vi "Show Cursors.vi"(6 "Cursor Options":T1={"font"={"Font Name"="Arial", "Size"=14, "Strikeout?"=FALSE, "Italic?"=FALSE, "Underline?"=FALSE, "Outline?"=FALSE, "Shadow?"=FALSE, "Bold?"=FALSE}, "size"=1, "Timestamp"=enum."at TOP", "Vertical Line?"=FALSE, "Horizontal Line?"=FALSE, "alignment(left, top)"={"horizontal"=enum."center", "vertical"=enum."center"}, "TextFormat"="%.3p %.3p %s", "time format (%H:%M:%S)"="%H:%M%:S"} {"size" min=1 max=50}, 8 "error in (no error)":errorcluster, 9 "Coords":T2, 10 "Graph Data":cluster{"Array":dbl[], "Array":dbl[]}[](array[cluster]), 11 "Grapg":refnum<vi>) -> (0 "error out":errorcluster, 3 "output picture":picture)   [LabVIEW 2019]
doc: "Shows real time cursors overlayed in a graph, using just one mouse move event case. The options for the cursors can be highly customized to set up a unique cursor style.\n\nUsage: Place this inside an event structure on any XY graph, in the \"Mouse Move\" event case. Set the options as an input cluster to override the defaults. The output picture control would typically be connected to the XY Graph's \"PlotImages.Front\" property item.\n\nCursor Options\n<b>Horizontal Line?</b> - Draws a horizontal line to intersect each plot\n<b>Verticle Line?</b> - Draws a verticle line at the mouse location to highlight the cursor location (typically on the time scale)\n<b>Timestamp</b> - Sets where to display the timestamp (if you want it at the top or bottom) Used best with the verticle line turned on.\n<b>Font</b> - Setup the font for displaying the cursor text\n<b>Alignment</b> - Sets the alignment options for the text relative to the cursor point\n<b>TextFormat</b> - Sets the text display format at the cursor points to show. Three input parameters are available for the text, which can be accessed using parameter numbers.\ninputs: \n1$ - Timestamp at cursor locations\n2$ - Value of the plot\n3$ - Name of the plot\n\nExamples: $2$.2f\\n\\n%1$s\nThis shows the value of the plot with 2 decimal places. A blank line, then the name of the plot"
uses:
  <vilib>/Utility/miscctls.llb/LVPoint32TypeDef.ctl
  controls/CursorOptions.ctl
panel:
  in  "input picture":picture
  # "%2$.2f\\n\\n%1$s"
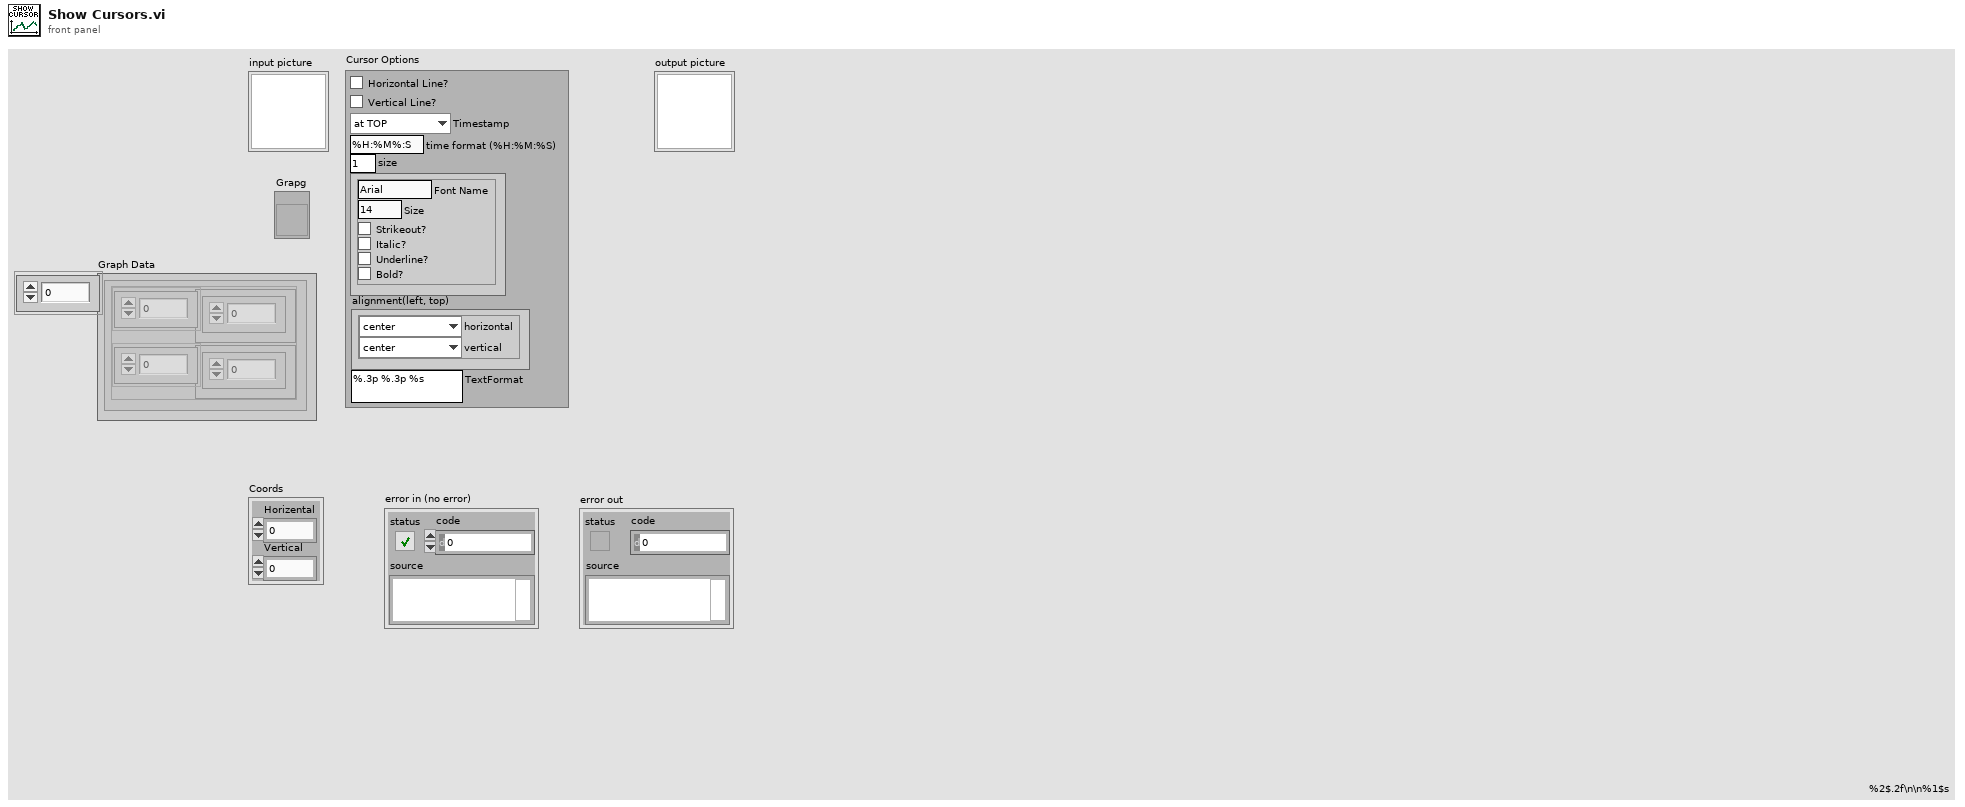
[diagram p1: front panel]
types:
  T1 = typedef "CursorOptions.ctl" = cluster{"font":cluster{"Font Name":string, "Size":i16, "Strikeout?":bool, "Italic?":bool, "Underline?":bool, "Outline?":bool, "Shadow?":bool, "Bold?":bool}, "size":i16, "Timestamp":enum16{"at TOP", "at BOTTOM", "none"}, "Vertical Line?":bool, "Horizontal Line?":bool, "alignment(left, top)":cluster{"horizontal":enum16{"left", "center", "right"}, "vertical":enum16{"top", "center", "bottom"}}, "TextFormat":string, "time format (%H:%M:%S)":string}
  T2 = typedef "LVPoint32TypeDef.ctl" = cluster{"Horizental":i32, "Vertical":i32}
  T3 = enum16{"User-specified Font", "Application Font", "System Font", "Dialog Font"}
  T4 = cluster{"horizontal":enum16{"left", "center", "right"}, "vertical":enum16{"top", "center", "bottom"}}
  T5 = cluster{"Font Name":string, "Size":i16, "Strikeout?":bool, "Italic?":bool, "Underline?":bool, "Outline?":bool, "Shadow?":bool, "Bold?":bool}
  T6 = typedef "LVRectTypeDef.ctl" = cluster{"Left":i16, "Top":i16, "Right":i16, "Bottom":i16}
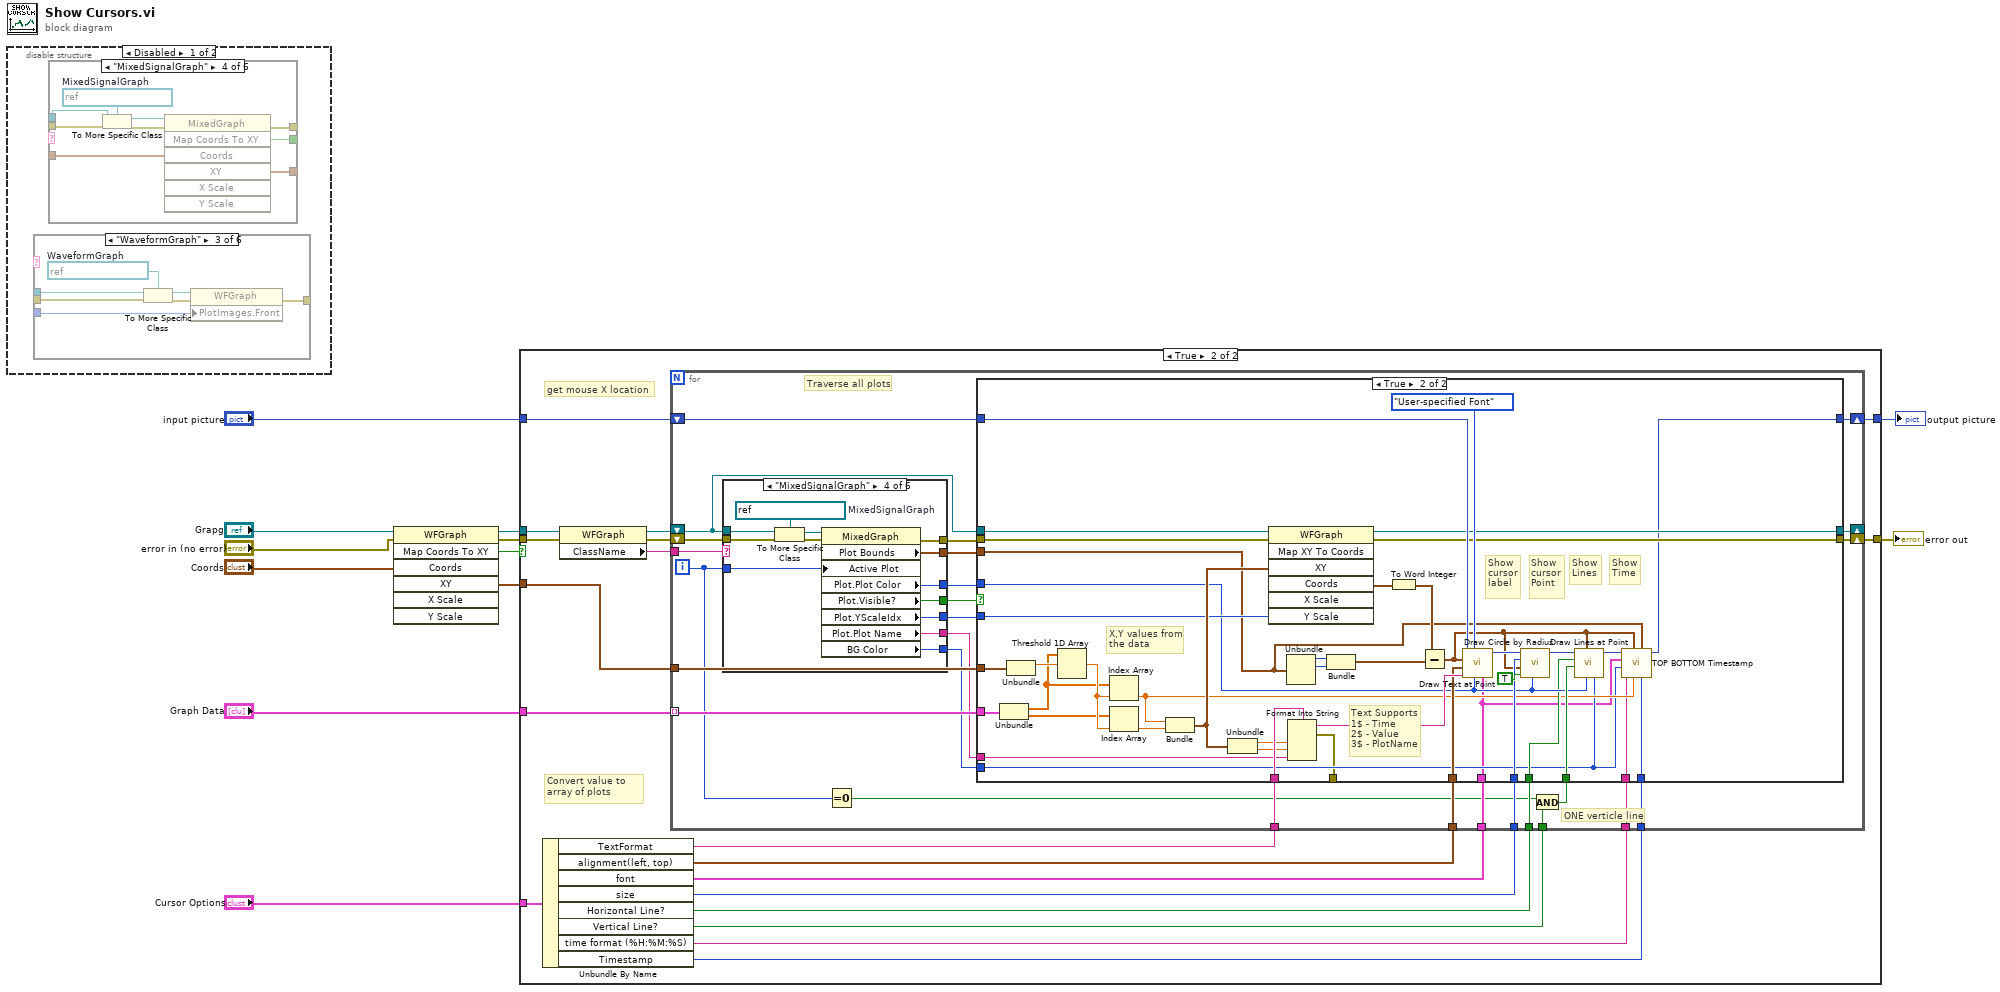
[diagram p0: block diagram]
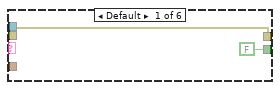
[diagram p2: hidden frame]
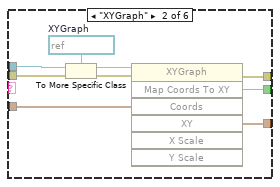
[diagram p3: hidden frame]
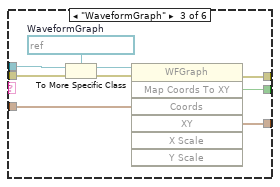
[diagram p4: hidden frame]
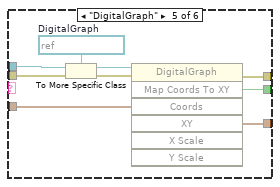
[diagram p5: hidden frame]
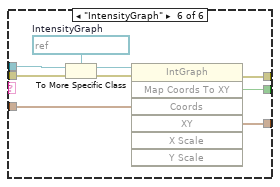
[diagram p6: hidden frame]
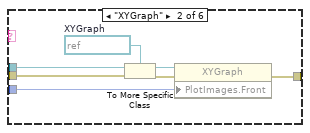
[diagram p8: hidden frame]
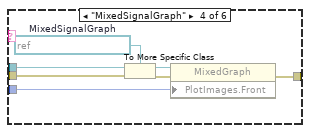
[diagram p9: hidden frame]
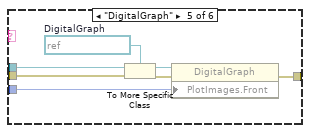
[diagram p10: hidden frame]
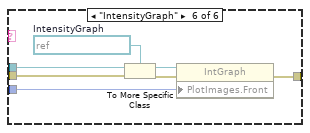
[diagram p11: hidden frame]
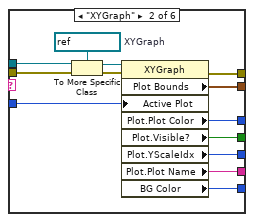
[diagram p15: hidden frame]
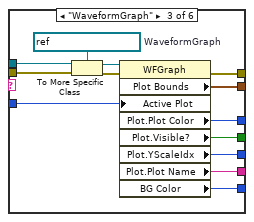
[diagram p16: hidden frame]
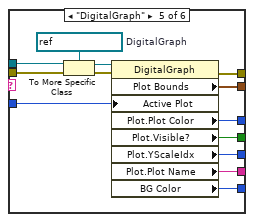
[diagram p17: hidden frame]
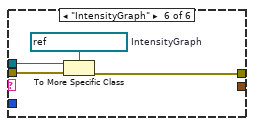
[diagram p18: hidden frame]
diagram:
  n1 = disable-structure shown="Disabled" {
    frame Disabled {
      n2 = case shown="\"WaveformGraph\"" {
        selector: _ -> [_ _ _ _ _ _]
        tunnel: _ -> [_ w67 w74 w81 w88 w95]
        tunnel: _ -> [w60 w65 w72 w76 w83 w90]
        tunnel: _ -> [_ w63 w68 w75 w82 w89]
        tunnel: [w60 w61 w70 w78 w85 w92] -> _
        frame Default {
        }
        frame "XYGraph" {
          w66 = refnum<vi> refnum  # XYGraph
          n3 = To More Specific Class(target class=w66, reference=w67, error in=w65) -> (specific class reference=w64:refnum<vi>, error out=w62:errorcluster)
          n4 = property class="XYGraph"(reference=w64, error in=w62, "PlotImages.Front"=w63) -> (error out=w61:errorcluster)  [unwired: 1 out]
        }
        frame "WaveformGraph" {
          w73 = refnum<vi> refnum  # WaveformGraph
          n5 = To More Specific Class(target class=w73, reference=w74, error in=w72) -> (specific class reference=w71:refnum<vi>, error out=w69:errorcluster)
          n6 = property class="WFGraph"(reference=w71, error in=w69, "PlotImages.Front"=w68) -> (error out=w70:errorcluster)  [unwired: 1 out]
        }
        frame "MixedSignalGraph" {
          w80 = refnum<vi> refnum  # MixedSignalGraph
          n7 = To More Specific Class(target class=w80, reference=w81, error in=w76) -> (specific class reference=w79:refnum<vi>, error out=w77:errorcluster)
          n8 = property class="MixedGraph"(reference=w79, error in=w77, "PlotImages.Front"=w75) -> (error out=w78:errorcluster)  [unwired: 1 out]
        }
        frame "DigitalGraph" {
          w87 = refnum<vi> refnum  # DigitalGraph
          n9 = To More Specific Class(target class=w87, reference=w88, error in=w83) -> (specific class reference=w86:refnum<vi>, error out=w84:errorcluster)
          n10 = property class="DigitalGraph"(reference=w86, error in=w84, "PlotImages.Front"=w82) -> (error out=w85:errorcluster)  [unwired: 1 out]
        }
        frame "IntensityGraph" {
          w94 = refnum<vi> refnum  # IntensityGraph
          n11 = To More Specific Class(target class=w94, reference=w95, error in=w90) -> (specific class reference=w93:refnum<vi>, error out=w91:errorcluster)
          n12 = property class="IntGraph"(reference=w93, error in=w91, "PlotImages.Front"=w89) -> (error out=w92:errorcluster)  [unwired: 1 out]
        }
      }
      n13 = case shown="\"MixedSignalGraph\"" {
        selector: _ -> [_ _ _ _ _ _]
        tunnel: _ -> [_ w23 w32 w41 w50 w59]
        tunnel: _ -> [w14 w21 w30 w39 w48 w57]
        tunnel: [w14 w20 w29 w37 w45 w54] -> _
        tunnel: _ -> [_ w16 w26 w35 w44 w52]
        tunnel: [_ w17 w24 w33 w43 w53] -> _
        tunnel: [FALSE ("Map Coords To XY") w15 w25 w34 w42 w51] -> _
        frame Default {
        }
        frame "XYGraph" {
          w22 = refnum<vi> refnum  # XYGraph
          n14 = To More Specific Class(target class=w22, reference=w23, error in=w21) -> (specific class reference=w19:refnum<vi>, error out=w18:errorcluster)
          n15 = invoke on="Invoke Node" class="XYGraph" method="Map Coords To XY"(reference=w19, error in=w18, "Coords"=w16) -> (error out=w20:errorcluster, "Map Coords To XY"=w15:bool, "XY"=w17:cluster{"X":dbl, "Y":dbl})  [unwired: 4 in, 4 out]
        }
        frame "WaveformGraph" {
          w31 = refnum<vi> refnum  # WaveformGraph
          n16 = To More Specific Class(target class=w31, reference=w32, error in=w30) -> (specific class reference=w28:refnum<vi>, error out=w27:errorcluster)
          n17 = invoke on="Invoke Node" class="WFGraph" method="Map Coords To XY"(reference=w28, error in=w27, "Coords"=w26) -> (error out=w29:errorcluster, "Map Coords To XY"=w25:bool, "XY"=w24:cluster{"X":dbl, "Y":dbl})  [unwired: 4 in, 4 out]
        }
        frame "MixedSignalGraph" {
          w40 = refnum<vi> refnum  # MixedSignalGraph
          n18 = To More Specific Class(target class=w40, reference=w41, error in=w39) -> (specific class reference=w38:refnum<vi>, error out=w36:errorcluster)
          n19 = invoke on="Invoke Node" class="MixedGraph" method="Map Coords To XY"(reference=w38, error in=w36, "Coords"=w35) -> (error out=w37:errorcluster, "Map Coords To XY"=w34:bool, "XY"=w33:cluster{"X":dbl, "Y":dbl})  [unwired: 4 in, 4 out]
        }
        frame "DigitalGraph" {
          w49 = refnum<vi> refnum  # DigitalGraph
          n20 = To More Specific Class(target class=w49, reference=w50, error in=w48) -> (specific class reference=w47:refnum<vi>, error out=w46:errorcluster)
          n21 = invoke on="Invoke Node" class="DigitalGraph" method="Map Coords To XY"(reference=w47, error in=w46, "Coords"=w44) -> (error out=w45:errorcluster, "Map Coords To XY"=w42:bool, "XY"=w43:cluster{"X":dbl, "Y":dbl})  [unwired: 4 in, 4 out]
        }
        frame "IntensityGraph" {
          w58 = refnum<vi> refnum  # IntensityGraph
          n22 = To More Specific Class(target class=w58, reference=w59, error in=w57) -> (specific class reference=w56:refnum<vi>, error out=w55:errorcluster)
          n23 = invoke on="Invoke Node" class="IntGraph" method="Map Coords To XY"(reference=w56, error in=w55, "Coords"=w52) -> (error out=w54:errorcluster, "Map Coords To XY"=w51:bool, "XY"=w53:cluster{"X":dbl, "Y":dbl})  [unwired: 4 in, 4 out]
        }
      }
    }
    frame Enabled {
    }
  }
  n24 = invoke on="Invoke Node" class="WFGraph" method="Map Coords To XY"(reference="Grapg", error in="error in (no error)", "Coords"="Coords") -> (reference out=w7:refnum<vi>, error out=w6:errorcluster, "Map Coords To XY"=w3:bool, "XY"=w4:cluster{"X":dbl, "Y":dbl})  [unwired: 4 in, 3 out]
  n25 = case shown="True" w3 {
    tunnel: w4 -> [_ w116]
    tunnel: w7 -> [_ w103]
    tunnel: [w96 w115] -> w10
    tunnel: w6 -> [w97 w99]
    tunnel: [w97 w114] -> w12
    tunnel: "input picture" -> [w96 w113]
    tunnel: "Cursor Options" -> [_ w105]
    tunnel: "Graph Data" -> [_ w98]
    frame False {
      # "not in plot area.  clear the image"
    }
    frame True {
      # "Convert value to array of plots"
      # "get mouse X location"
      n26 = Unbundle By Name(w105) -> ("TextFormat"=w112:string, "alignment(left, top)"=w111:T4, "font"=w110:T5, "size"=w109:i16, "Horizontal Line?"=w108:bool, "Vertical Line?"=w107:bool, "time format (%H:%M:%S)"=w104:string, "Timestamp"=w106:enum16{"at TOP", "at BOTTOM", "none"})
      n27 = property class="WFGraph"(reference=w103, error in=w99) -> (reference out=w102:refnum<vi>, error out=w100:errorcluster, "ClassName"=w101:string)
      n28 = for {
        tunnel: w98 -> [w129] mode=indexing
        shift-right: [w143] -> _
        shift-left: w102 -> [w118]
        tunnel: w116 -> [w130]
        shift-right: [w141] -> w115
        shift-left: w113 -> [w142]
        shift-right: [w140] -> w114
        shift-left: w100 -> [w126]
        tunnel: w109 -> [w139]
        tunnel: w111 -> [w138]
        tunnel: w110 -> [w137]
        tunnel: w112 -> [w136]
        tunnel: w108 -> [w135]
        tunnel: w107 -> [w132]
        tunnel: w106 -> [w131]
        tunnel: w104 -> [w128]
        tunnel: w101 -> [w117]
        i -> [w127]
        # "Traverse all plots"
        # "ONE verticle line"
        n29 = case shown="\"MixedSignalGraph\"" w117 {
          tunnel: w118 -> [_ w157 w170 w183 w196 w200]
          tunnel: w126 -> [w144 w155 w168 w181 w194 w198]
          tunnel: [w144 w153 w165 w178 w191 w197] -> w120
          tunnel: w127 -> [_ w151 w163 w172 w190 _]
          tunnel: [_ w150 w162 w173 w189 _] -> w121
          tunnel: [_ w149 w161 w174 w188 _] -> w122
          tunnel: [_ w148 w160 w175 w187 _] -> w123
          tunnel: [_ w147 w164 w171 w184 _] -> w119
          tunnel: [_ w146 w159 w176 w186 _] -> w125
          tunnel: [_ w145 w158 w177 w185 _] -> w124
          frame Default {
          }
          frame "XYGraph" {
            w156 = refnum<vi> refnum  # XYGraph
            n30 = To More Specific Class(target class=w156, reference=w157, error in=w155) -> (specific class reference=w154:refnum<vi>, error out=w152:errorcluster)
            n31 = property on="Property Node" class="XYGraph"(reference=w154, error in=w152, "Active Plot"=w151) -> (error out=w153:errorcluster, "Plot Bounds"=w147:T6, "Plot.Plot Color"=w150:u32, "Plot.Visible?"=w149:bool, "Plot.YScaleIdx"=w148:u32, "Plot.Plot Name"=w146:string, "BG Color"=w145:u32)  [unwired: 1 out]
          }
          frame "WaveformGraph" {
            w169 = refnum<vi> refnum  # WaveformGraph
            n32 = To More Specific Class(target class=w169, reference=w170, error in=w168) -> (specific class reference=w167:refnum<vi>, error out=w166:errorcluster)
            n33 = property on="Property Node" class="WFGraph"(reference=w167, error in=w166, "Active Plot"=w163) -> (error out=w165:errorcluster, "Plot Bounds"=w164:T6, "Plot.Plot Color"=w162:u32, "Plot.Visible?"=w161:bool, "Plot.YScaleIdx"=w160:u32, "Plot.Plot Name"=w159:string, "BG Color"=w158:u32)  [unwired: 1 out]
          }
          frame "MixedSignalGraph" {
            w182 = refnum<vi> refnum  # MixedSignalGraph
            n34 = To More Specific Class(target class=w182, reference=w183, error in=w181) -> (specific class reference=w180:refnum<vi>, error out=w179:errorcluster)
            n35 = property on="Property Node" class="MixedGraph"(reference=w180, error in=w179, "Active Plot"=w172) -> (error out=w178:errorcluster, "Plot Bounds"=w171:T6, "Plot.Plot Color"=w173:u32, "Plot.Visible?"=w174:bool, "Plot.YScaleIdx"=w175:u32, "Plot.Plot Name"=w176:string, "BG Color"=w177:u32)  [unwired: 1 out]
          }
          frame "DigitalGraph" {
            w195 = refnum<vi> refnum  # DigitalGraph
            n36 = To More Specific Class(target class=w195, reference=w196, error in=w194) -> (specific class reference=w193:refnum<vi>, error out=w192:errorcluster)
            n37 = property on="Property Node" class="DigitalGraph"(reference=w193, error in=w192, "Active Plot"=w190) -> (error out=w191:errorcluster, "Plot Bounds"=w184:T6, "Plot.Plot Color"=w189:u32, "Plot.Visible?"=w188:bool, "Plot.YScaleIdx"=w187:u32, "Plot.Plot Name"=w186:string, "BG Color"=w185:u32)  [unwired: 1 out]
          }
          frame "IntensityGraph" {
            w199 = refnum<vi> refnum  # IntensityGraph
            n38 = To More Specific Class(target class=w199, reference=w200, error in=w198) -> (error out=w197:errorcluster)  [unwired: 1 out]
          }
        }
        n39 = Equal To 0?(x=w127) -> (x = 0?=w133:bool)
        n40 = And(x=w133, y=w132) -> (x .and. y?=w134:bool)
        n41 = case shown="True" w122 {
          tunnel: w119 -> [_ w212]
          tunnel: [w203 w206] -> w143
          tunnel: w129 -> [_ w237]
          tunnel: w130 -> [_ w236]
          tunnel: w142 -> [w202 w235]
          tunnel: w118 -> [w203 w232]
          tunnel: [w202 w204] -> w141
          tunnel: w121 -> [_ w221]
          tunnel: w120 -> [w201 w228]
          tunnel: [w201 w205] -> w140
          tunnel: w123 -> [_ w227]
          tunnel: w139 -> [_ w226]
          tunnel: w138 -> [_ w225]
          tunnel: w137 -> [_ w210]
          tunnel: w136 -> [_ w224]
          tunnel: w135 -> [_ w220]
          tunnel: w134 -> [_ w223]
          tunnel: w125 -> [_ w217]
          tunnel: w131 -> [_ w214]
          tunnel: w124 -> [_ w211]
          tunnel: [_ w208] -> _
          tunnel: w128 -> [_ w207]
          frame False {
            # "plot is not visible, so don't show the cursor for it."
          }
          frame True {
            # "Show\nTime"
            # "Show\nLines"
            # "Show\ncursor\nPoint"
            # "Show\ncursor\nlabel"
            # "Text Supports\n1$ - Time\n2$ - Value\n3$ - PlotName"
            # "X,Y values from the data"
            n42 = Unbundle(w237) -> ("Array"=w209:dbl[], "Array"=w239:dbl[])
            n43 = Unbundle(w236) -> ("X"=w238:dbl)  [unwired: 1 out]
            n44 = Threshold 1D Array(2:w238, 3:w209) -> (0:w240:dbl)  [unwired: 1 in]
            n45 = Index Array(array=w209, index=w240) -> (element=w215:dbl)
            n46 = Index Array(array=w239, index=w240) -> (element=w241:dbl)
            n47 = Bundle("X"=w215, "X"=w241) -> (w234:cluster{"X":dbl, "X":dbl})  [unwired: 1 in]
            n48 = Unbundle(w234) -> ("X"=w219:dbl, "X"=w218:dbl)
            n49 = invoke on="Invoke Node" class="WFGraph" method="Map XY To Coords"(reference=w232, error in=w228, "XY"=w234, "Y Scale"=w227) -> (reference out=w206:refnum<vi>, error out=w205:errorcluster, "Coords"=w246:T2)  [unwired: 3 in, 4 out]
            n50 = Unbundle(w212) -> ("Left"=w244:i16, "Top"=w245:i16)  [unwired: 2 out]
            n51 = Format Into String(format string=w224, w219, w218, w217) -> (resulting string=w233:string, error out=w208:errorcluster)  [unwired: 2 in]
            n52 = Bundle("Left"=w244, "Top"=w245) -> (w242:cluster{"Left":i16, "Top":i16})  [unwired: 1 in]
            n53 = To Word Integer(number=w246) -> (16bit integer=w243:cluster{"Horizontal":i16, "Vertical":i16})
            n54 = Subtract(x=w243, y=w242) -> (x-y=w213:cluster{i16, i16})
            n55 = call <vilib>:"Draw Text at Point.vi"("[user-specified font]"=w210, "text color(black)"=w221, "desired font(Application)"=T3."User-specified Font", "text"=w233, "alignment(left, top)"=w225, "origin"=w213, "picture"=w235) -> ("new picture"=w231:picture)  [unwired: 3 in, 1 out]
            n56 = call <vilib>:"Draw Circle by Radius.vi"("color(black)"=w221, "fill?(F)"=TRUE, "pixel center"=w213, "radius"=w226, "picture"=w231) -> ("new picture"=w222:picture)  [unwired: 6 in]
            n57 = call "Draw Lines at Point.vi"("GraphBGK"=w211, "color(black)"=w221, "pixel center"=w213, "Vertical Line?"=w223, "Horizontal Line?"=w220, "new picture in"=w222) -> ("new picture out"=w216:picture)  [unwired: 5 in]
            n58 = call "TOP BOTTOM Timestamp.vi"("Format"=w214, "Rect"=w212, "Timestamp"=w215, "pixel center"=w213, "time format (%H:%M:%S)"=w207, "GraphBGK"=w211, "font"=w210, "new picture in"=w216) -> ("new picture out"=w204:picture)  [unwired: 3 in]
          }
        }
      }
    }
  }
  "error out" <- w12
  "output picture" <- w10
